vi "Binary.vi"(8 "Error In":errorcluster) -> (0 "Error Out":errorcluster)   [LabVIEW 2017, in "Tests.lvlib" / "From Msgpack.lvlib"]
uses:
  From Msgpack.lvlib
  <vilib>/addons/_JKI Toolkits/Caraya/classes/Test/Test.lvclass
  src/LabPack/LabPack.lvlib
  <vilib>/addons/_JKI Toolkits/Caraya/classes/Assert/Assert.lvclass
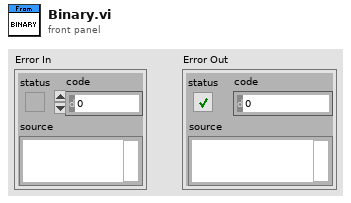
[diagram p1: front panel]
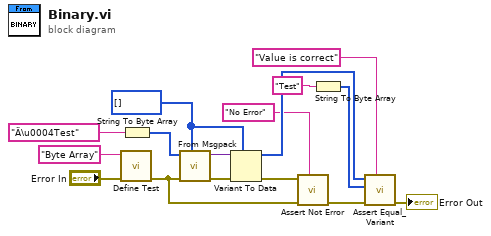
[diagram p0: block diagram]
diagram:
  w3 = u8[] []
  n1 = call <vilib>:"Define Test.vi"("error in (no error)"="Error In", "Label (VI Title)"="Byte Array") -> ("error out"=w10:errorcluster)  [unwired: 9 in]
  n2 = String To Byte Array(string="Ä\u0004Test") -> (unsigned byte array=w13:u8[])
  n3 = call "From Msgpack.vi"("Types and Defaults"=w3, "Error In"=w10, "Msgpack Data"=w13) -> ("Error Out"=w14:errorcluster, "Value"=w12:variant)  [unwired: 7 in]
  n4 = Variant To Data(error in=w14, type=w3, Variant=w12) -> (data=w7:u8[], error out=w11:errorcluster)
  n5 = call <vilib>:"Assert Not Error.vi"("Label"="No Error", "error in (no error)"=w10, "Not Error?"=w11) -> ("error out"=w9:errorcluster)  [unwired: 8 in]
  n6 = String To Byte Array(string="Test") -> (unsigned byte array=w1:u8[])
  n7 = call <vilib>:"Assert Equal_Variant.vi"("Label"="Value is correct", "error in (no error)"=w9, "Y"=w1, "X"=w7) -> ("error out"=→"Error Out":errorcluster)  [unwired: 7 in]
